vi "Low pass filter.vi"(0 "error in (no error)":errorcluster, 2 "data":waveform(dbl)[](array[waveform]), 3 "Lock-in settings":T1={"Sine Frequency, Hz"=0.0, "Time constant, s"=0.12500000000000006, "Low-pass filter"=enum."No filtering", "Output representation"=enum."Real/Imaginary", "Phases, deg"=[], "Low-pass filter Order"=1, "Decimating factor"=1, "Samples to Read"=10000, "Post-filter decimation"=1, "Blocks to average"=1, "Trig delay, points"=0, "Harmonics per channel"=[], "Amplitude scale"=enum."RMS"} {"Time constant, s" format="%.1e"}, 5 "Initialize?":bool) -> (8 "error out":errorcluster, 10 "signal(s) out":waveform(dbl)[](array[waveform]), 11 "Lock-in settings out":T1={"Sine Frequency, Hz"=0.0, "Time constant, s"=0.12500000000000006, "Low-pass filter"=enum."No filtering", "Output representation"=enum."Real/Imaginary", "Phases, deg"=[], "Low-pass filter Order"=1, "Decimating factor"=1, "Samples to Read"=10000, "Post-filter decimation"=1, "Blocks to average"=1, "Trig delay, points"=0, "Harmonics per channel"=[], "Amplitude scale"=enum."RMS"} {"Time constant, s" format="%.1e"})   [LabVIEW 2015]
uses:
  Controls/Lockin Settings.ctl
  Controls/Harmonics per channel.ctl
  <vilib>/measure/macond.llb/IIR Filter for N Chan.vi
  <vilib>/measure/NI_MAPro.lvlib
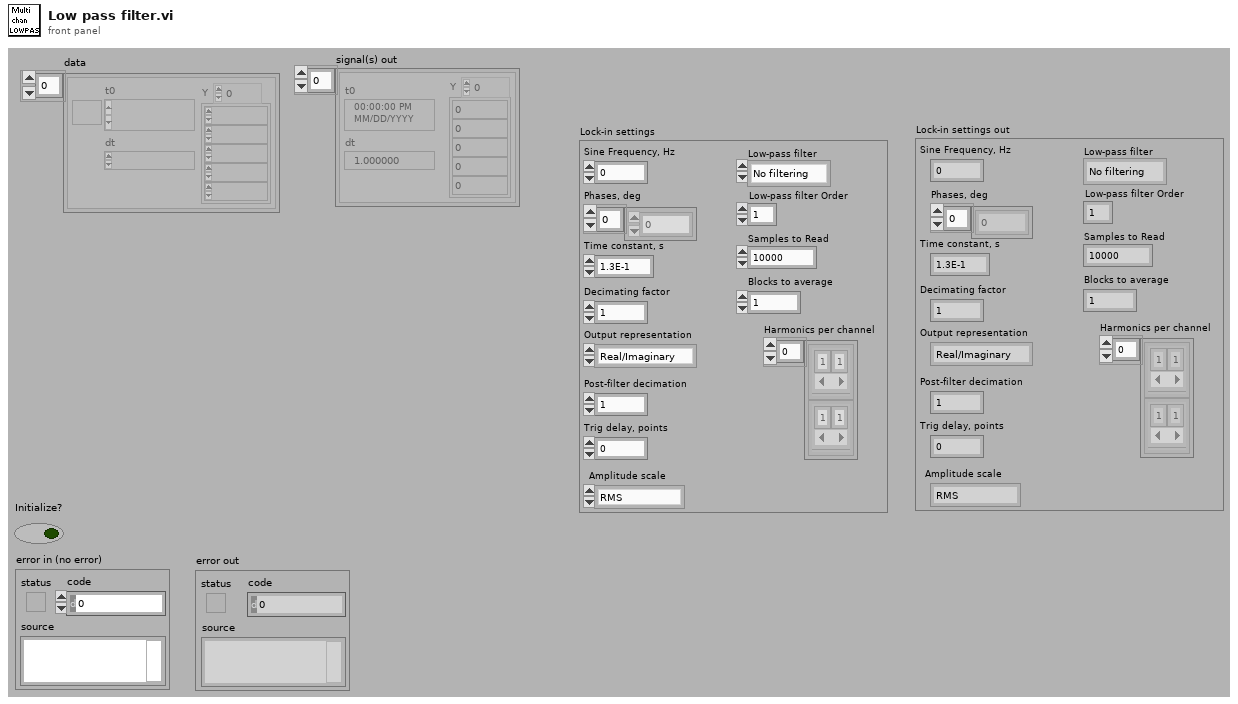
[diagram p1: front panel]
types:
  T1 = typedef "Lockin Settings.ctl" = cluster{"Sine Frequency, Hz":dbl, "Time constant, s":dbl, "Low-pass filter":enum16{"No filtering", "Butterworth", "Bessel"}, "Output representation":enum16{"Real/Imaginary", "Polar"}, "Phases, deg":dbl[], "Low-pass filter Order":i32, "Decimating factor":i32, "Samples to Read":i32, "Post-filter decimation":i32, "Blocks to average":i32, "Trig delay, points":i32, "Harmonics per channel":T2, "Amplitude scale":enum16{"Amplitude", "RMS", "Peak-to-Peak"}}
  T2 = typedef "Harmonics per channel.ctl" = cluster{"Harmonics":i32[]}[]
  T3 = enum16{"Lowpass", "Highpass", "Bandpass", "Bandstop"}
  T4 = enum16{"Off", "Butterworth", "Chebyshev", "Inverse Chebyshev", "Elliptic", "Bessel"}
  T5 = cluster{"Topology":enum16{"Off", "Butterworth", "Chebyshev", "Inverse Chebyshev", "Elliptic", "Bessel"}, "Type":enum16{"Lowpass", "Highpass", "Bandpass", "Bandstop"}, "Low-pass filter Order":i32, dbl, dbl, "PB Ripple":dbl, "SB Attenuation":dbl}
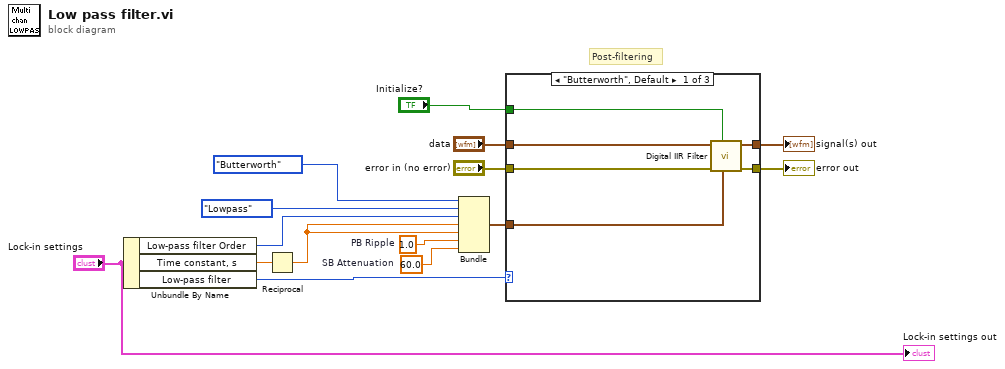
[diagram p0: block diagram]
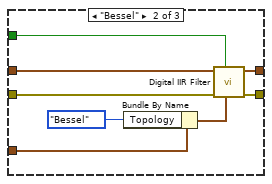
[diagram p2: hidden frame]
diagram:
  w9 = 60.0  # SB Attenuation
  w10 = 1.0  # PB Ripple
  # "Post-filtering"
  n1 = Unbundle By Name("Lock-in settings") -> ("Low-pass filter Order"=w6:i32, "Time constant, s"=w5:dbl, "Low-pass filter"=w3:enum16{"No filtering", "Butterworth", "Bessel"})
  n2 = Reciprocal(x=w5) -> (1/x=w8:dbl)
  n3 = Bundle("Topology"=T4."Butterworth", "Type"=T3."Lowpass", "Low-pass filter Order"=w6, w8, w8, "PB Ripple"=w10, "SB Attenuation"=w9) -> (w4:T5)  [unwired: 1 out]
  n4 = case shown="\"Butterworth\", Default" w3 {
    tunnel: "Initialize?" -> [w20 w28 _]
    tunnel: "data" -> [w18 w26 w31]
    tunnel: [w19 w27 w31] -> w14
    tunnel: [w21 w29 w30] -> w15
    tunnel: "error in (no error)" -> [w17 w25 w30]
    tunnel: w4 -> [w16 w24 _]
    frame "Butterworth", Default {
      n5 = call-poly <vilib>:"Digital IIR Filter.vi"("IIR filter specifications"=w16, "reset filters"=w20, "error in (no error)"=w17, "signal(s) in"=w18) -> ("error out"=w21:errorcluster, "signal(s) out"=w19:waveform(dbl)[])  [unwired: 2 in, 4 out]
    }
    frame "Bessel" {
      n6 = Bundle By Name(cluster=w24, "Topology"=T4."Bessel") -> (w23:T5)
      n7 = call-poly <vilib>:"Digital IIR Filter.vi"("IIR filter specifications"=w23, "reset filters"=w28, "error in (no error)"=w25, "signal(s) in"=w26) -> ("error out"=w29:errorcluster, "signal(s) out"=w27:waveform(dbl)[])  [unwired: 2 in, 4 out]
    }
    frame "No filtering" {
    }
  }
  "signal(s) out" <- w14
  "error out" <- w15
  "Lock-in settings out" <- "Lock-in settings"
